vi "Configure Dialog.vi"(8 "error in (no error)":errorcluster, 11 "Configure Sample Rate [ARB] Msg in":refnum<class "Configure Sample Rate [ARB] Msg.lvclass">) -> (0 "error out":errorcluster, 2 "Ok?":bool, 3 "Configure Sample Rate [ARB] Msg out":refnum<class "Configure Sample Rate [ARB] Msg.lvclass">)   [LabVIEW 2014, in "CS++Fgen.lvlib" / "Configure Sample Rate [ARB] Msg.lvclass"]
uses:
  Configure Sample Rate [ARB] Msg.lvclass
  Configure Sample Rate [ARB] Msg.lvclass/Configure Sample Rate [ARB] Msg.ctl
panel:
  in  "sample rate (1000 Samp/s)":dbl[unit]=1000.0 caption="Sample Rate" format="%^.2e"
  in  "OK Button":bool
  in  "Cancel Button":bool
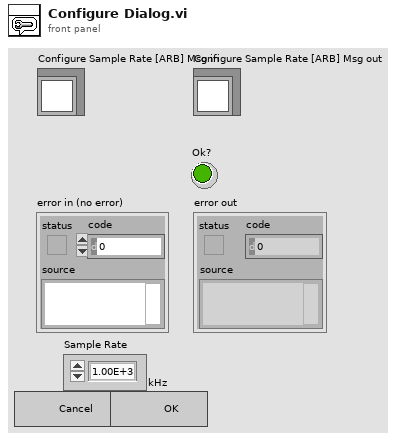
[diagram p1: front panel]
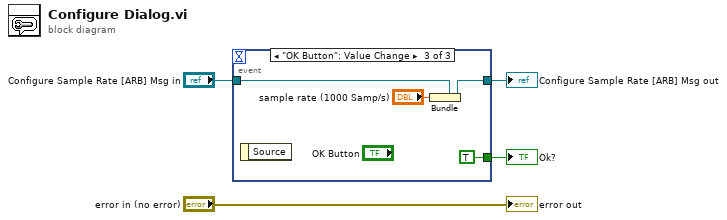
[diagram p0: block diagram]
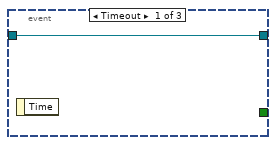
[diagram p2: hidden frame]
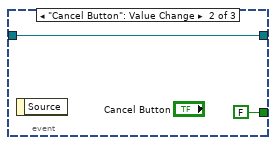
[diagram p3: hidden frame]
diagram:
  n1 = event shown="[2] \"OK Button\": Value Change" {
    selector: _ -> [_ _ _]
    dyn-events: _ -> [_ _ _]
    timeout: _ -> [_ _ _]
    tunnel: [w5 w7 w9] -> w3
    tunnel: "Configure Sample Rate [ARB] Msg in" -> [w5 w7 w11]
    tunnel: [_ FALSE TRUE] -> w1
    event Timeout {
      n2 = event-data() -> ()  [unwired: 1 in, 1 out]
    }
    event "Cancel Button": Value Change {
      n3 = event-data() -> ()  [unwired: 1 in, 1 out]
    }
    event "OK Button": Value Change {
      n4 = event-data() -> ()  [unwired: 1 in, 1 out]
      n5 = Bundle(cluster=w11, "sample rate (1000 Samp/s)") -> (w9:refnum<class "Configure Sample Rate [ARB] Msg.lvclass">)
    }
  }
  "Configure Sample Rate [ARB] Msg out" <- w3
  "Ok?" <- w1
  "error out" <- "error in (no error)"
